vi "Dispatch Worker Mode Example(Async).vi"() -> ()   [LabVIEW 2014]
uses:
  user.lib/_NEVSTOP/JKI State Machine ++/_Support/JKISMQ/_JKISMQFGV.vi
  user.lib/_NEVSTOP/JKI State Machine ++/JKI-State-Machine-Plus.lvlib
panel:
  in  "Macro: Exit -@ Worker":bool
  in  "DoSth: DoA -@ Worker":bool
  in  "Name(\"\" to use uuid)":string="Event JKISM"
  out "State History":string
  in  "DoSth: DoA -> Worker":bool
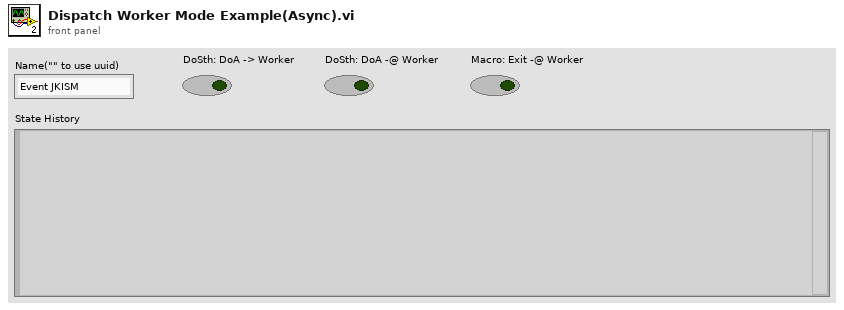
[diagram p1: front panel]
types:
  T1 = enum32{"Invalid", "Standard", "Closed", "Hidden", "Minimized", "Maximized"}
  T2 = enum32{"invalid app kind", "Development System", "Run Time System", "Student Edition", "Embedded LabVIEW", "Evaluation", "Custom"}
  T3 = cluster{"Core":cluster{"Current VI Reference":refnum<vi>, "Close Panel on Exit?":bool}, "Your Boolean data":bool, "Your string data":string}
  T4 = cluster{"Current VI Reference":refnum<vi>, "Close Panel on Exit?":bool}
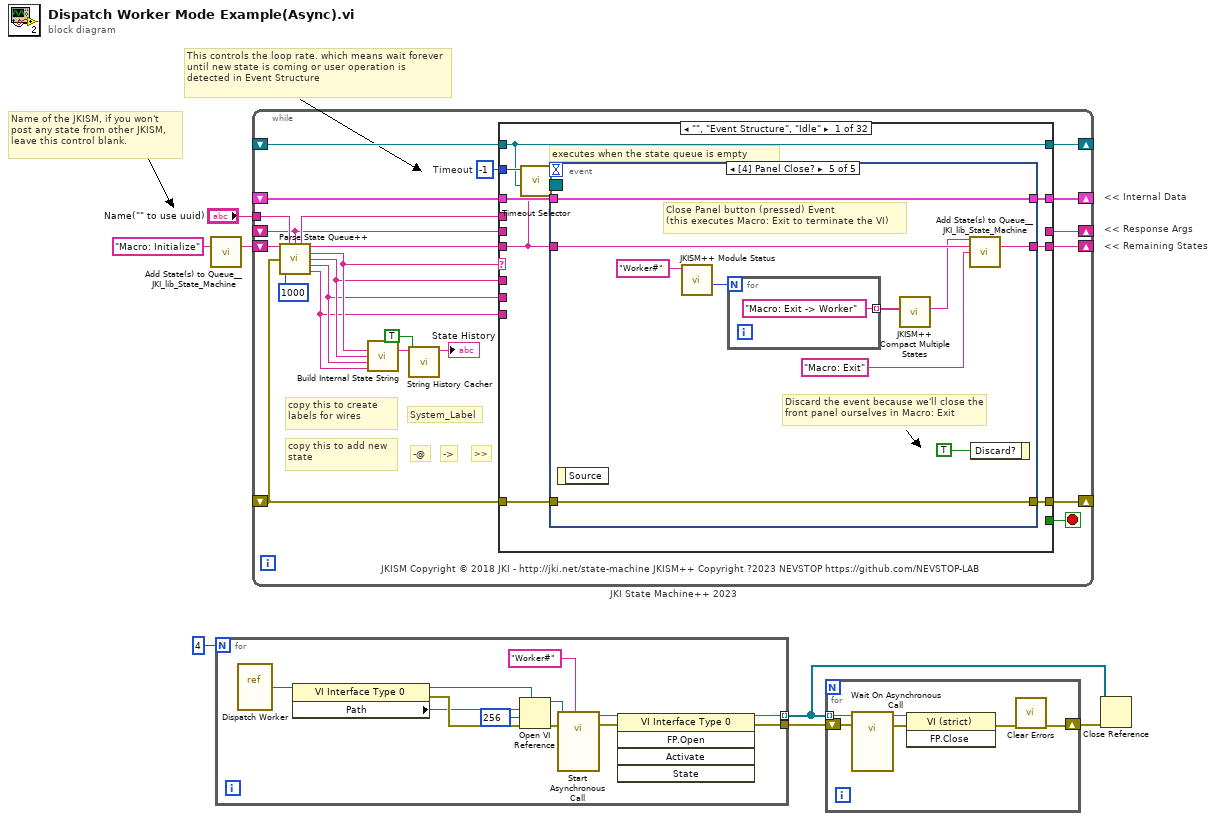
[diagram p0: block diagram]
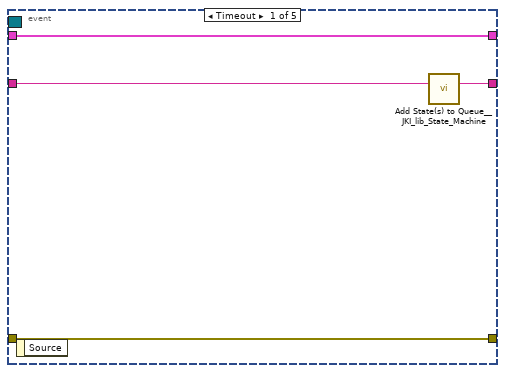
[diagram p2: hidden frame]
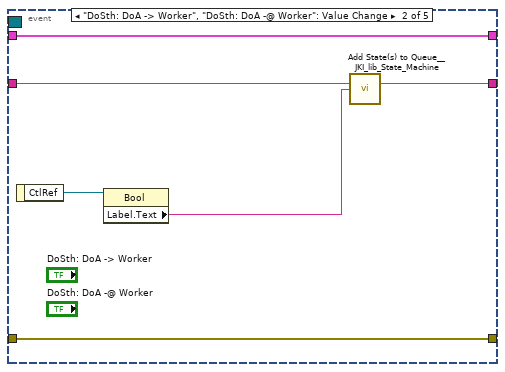
[diagram p3: hidden frame]
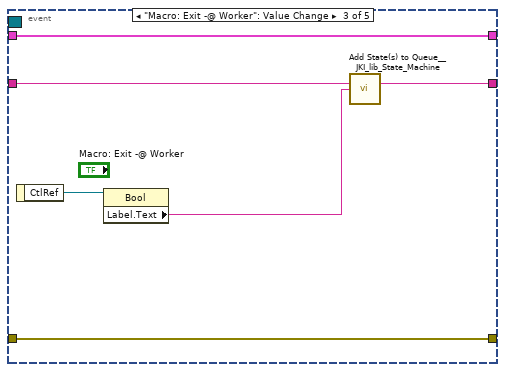
[diagram p4: hidden frame]
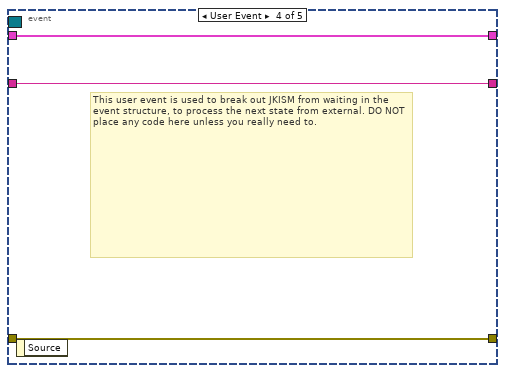
[diagram p5: hidden frame]
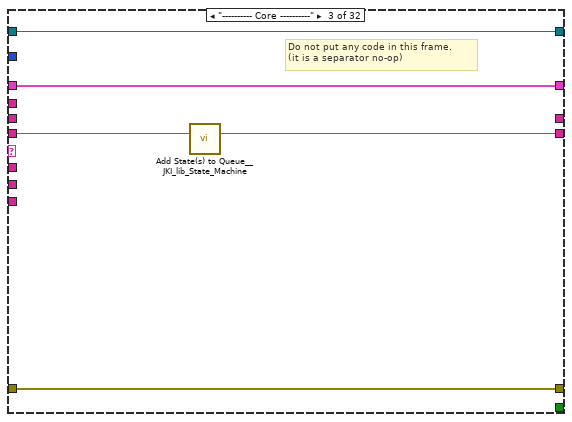
[diagram p7: hidden frame]
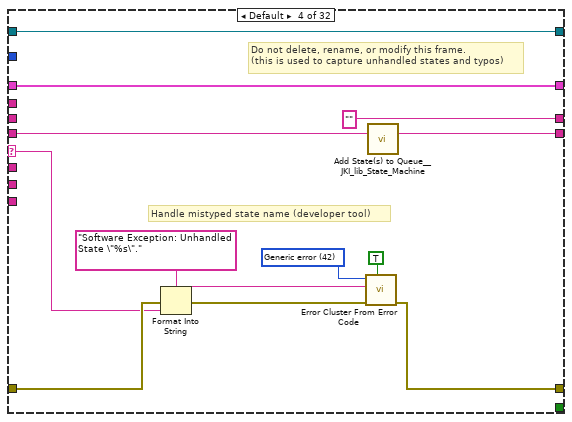
[diagram p8: hidden frame]
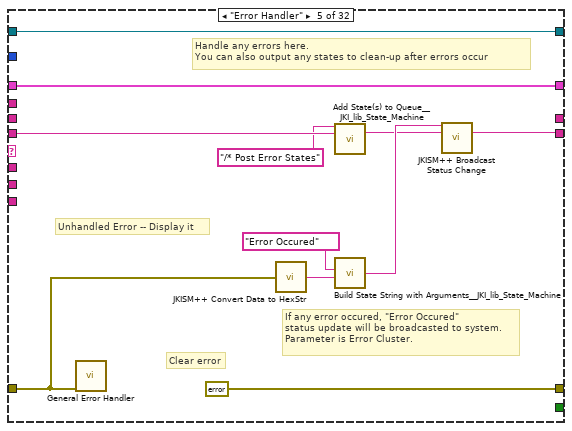
[diagram p9: hidden frame]
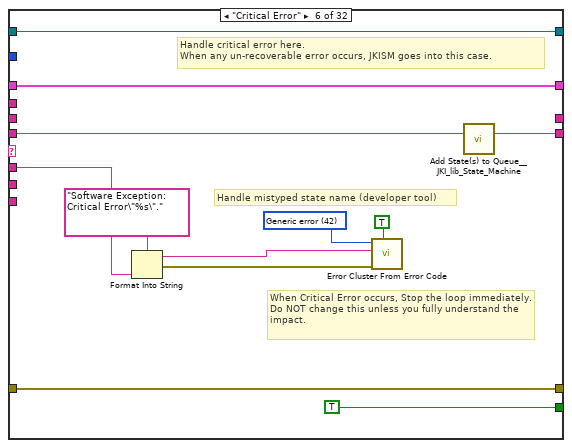
[diagram p10: hidden frame]
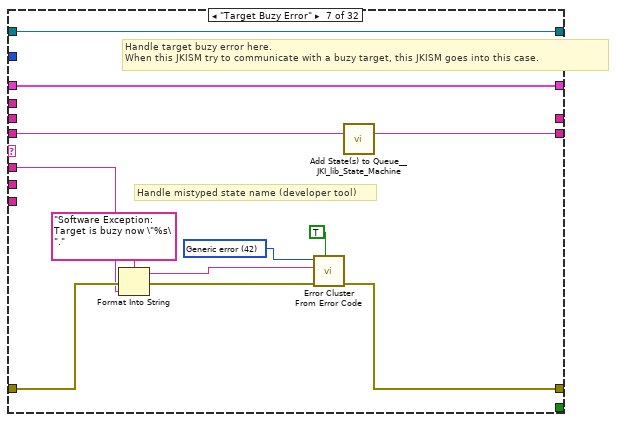
[diagram p11: hidden frame]
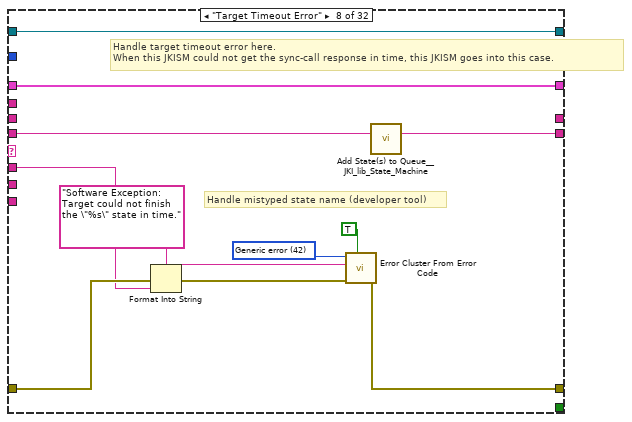
[diagram p12: hidden frame]
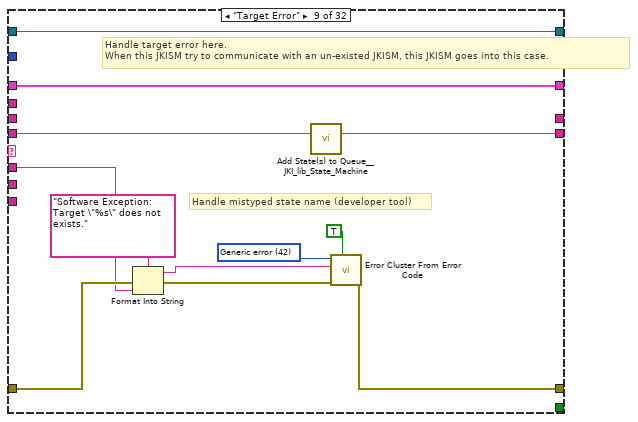
[diagram p13: hidden frame]
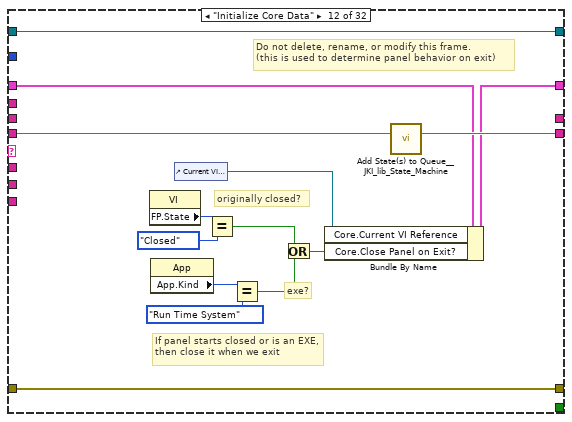
[diagram p16: hidden frame]
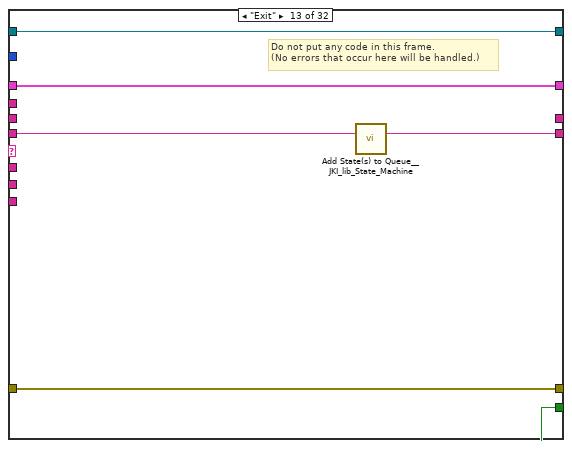
[diagram p17: hidden frame]
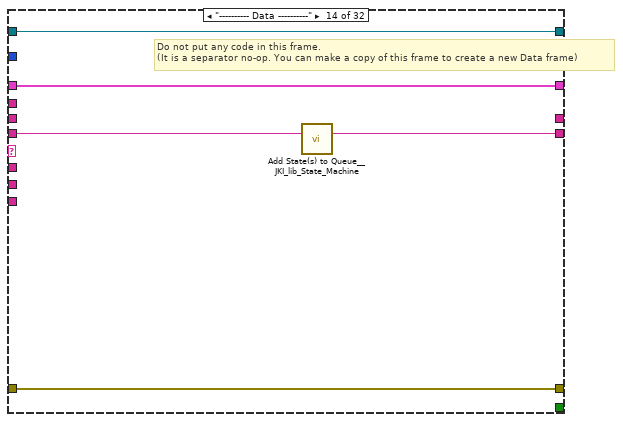
[diagram p18: hidden frame]
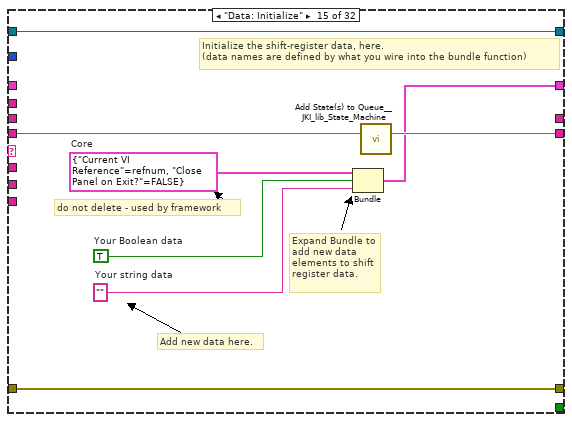
[diagram p19: hidden frame]
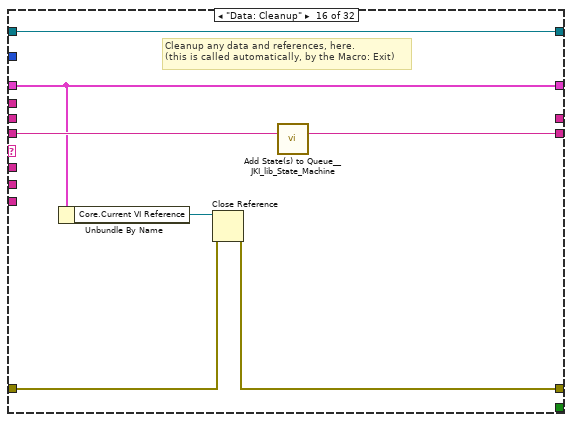
[diagram p20: hidden frame]
diagram:
  # "Name of the JKISM, if you won't post any state from other JKISM,  leave this control blank."
  # "This controls the loop rate. which means wait forever until new state is coming or user operation is detected in Event Structure"
  # "<< Internal Data"
  # "<< Response Args"
  # "<< Remaining States"
  n1 = call <vilib>:"Add State(s) to Queue__JKI_lib_State_Machine.vi"("State(s) in (\"\")"="Macro: Initialize") -> ("States Out"=w7:string)  [unwired: 14 in]
  n2 = for {
    N: 4 -> [_]
    tunnel: [w9] -> w4
    tunnel: [w10] -> w1 mode=indexing
    n3 = vi-ref "Dispatch Worker.vi"() -> (w13:refnum<vi>)
    n4 = property class="VI Interface Type 0"(reference=w13) -> (reference out=w17:refnum<vi>, error out=w15:errorcluster, "Path"=w14:path)  [unwired: 1 in]
    n5 = Open VI Reference(type specifier VI Refnum (for type only)=w17, vi path=w14, options=256, error in (no error)=w15) -> (vi reference=w16:refnum<vi>, error out=w12:errorcluster)  [unwired: 2 in]
    n6 = call-by-ref "Start Asynchronous Call"(reference=w16, error in=w12, "Name(\"\" to use uuid)"="Worker#" ("Name(\"\" to use uuid)")) -> (reference out=w11:refnum<vi>, error out=w8:errorcluster)  [unwired: 11 in]
    n7 = invoke class="VI Interface Type 0" method="FP.Open"(reference=w11, error in=w8) -> (reference out=w10:refnum<vi>, error out=w9:errorcluster)  [unwired: 3 in, 3 out]
  }
  n8 = while "JKI State Machine++ 2023" {
    shift-right: [w37] -> _
    shift-left: _ -> [w36]
    shift-right: [w40] -> _
    shift-left: _ -> [w34]
    shift-right: [w39] -> _
    shift-left: w7 -> [w41]
    tunnel: "Name(\"\" to use uuid)" -> [w29]
    shift-right: [w32] -> _
    shift-left: _ -> [w21]
    shift-right: [w31] -> _
    shift-left: _ -> [w30]
    stop <- w38 stop-if-true
    w35 = -1  # Timeout
    # "JKISM Copyright © 2018 JKI - http://jki.net/state-machine JKISM++ Copyright ?2023 NEVSTOP https://github.com/NEVSTOP-LAB"
    # "copy this to add new state"
    # ">>"
    # "->"
    # "-@"
    # "copy this to create labels for wires"
    # "System_Label"
    n9 = call "Parse State Queue++.vi"("State Queue"=w41, "Name(\"\" to use uuid)"=w29, "Response Arguments"=w21, "Error In (no error)"=w34, "Response Timeout(5000ms)"=1000 ("Response Timeout(1000ms)")) -> ("Name Used"=w22:string, "Remaining States"=w42:string, "Current State"=w26:string, "Arguments"=w25:string, "Argument - State"=w24:string, "From Who"=w23:string)  [unwired: 5 in]
    n10 = call "Build Internal State String.vi"("State"=w26, "Arguments (\"\")"=w25, "Arg-State (\"\")"=w24, "Source (\"\")"=w23) -> ("State with Arguments"=w27:string)  [unwired: 11 in]
    n11 = call "String History Cacher.vi"("Include Timestamp(F)"=TRUE, "String"=w27) -> ("String Cache"=→"State History":string)  [unwired: 9 in]
    n12 = case shown="\"\", \"Event Structure\", \"Idle\"" w26 {
      selector: w26 -> [_ _ _ w93 _ _ _ _ _ _ _ _ _ _ _ _ _ _ _ _ _ _ _ _ _ _ _ _ _ _ _ _]
      tunnel: w42 -> [w43 w84 w90 w97 w114 w124 w127 w144 w156 w165 w169 w184 w190 w195 w203 w210 w215 w221 w225 w231 w236 w243 w259 w329 w335 w346 w349 w354 w360 w368 w374 w380]
      tunnel: w25 -> [_ _ _ _ _ w117 w129 w140 w152 _ _ _ _ _ _ _ _ _ _ _ _ w238 w253 _ _ _ _ _ w357 _ _ _]
      tunnel: w36 -> [w50 w83 w87 w95 w112 w125 w131 w142 w154 w164 w168 w177 w188 w192 _ w205 w212 w220 w224 w228 w234 w241 w255 w326 w332 w343 w348 w353 w359 w365 w371 w377]
      tunnel: [w49 w85 w88 w99 errorcluster {"status"=FALSE, "code"=0, "source"=""} ("error out") w126 w134 w146 w158 w166 w170 w181 w187 w193 w200 w206 w213 w216 w223 w229 w233 w239 w256 w327 w333 w344 w350 w355 w361 w366 w372 w378] -> w40
      tunnel: w34 -> [w48 w85 w88 w98 w104 w126 w133 w145 w157 w166 w170 w181 w187 w193 w200 w207 w213 _ w226 w229 w233 w240 w257 w327 w333 w344 w350 w355 w361 w366 w372 w378]
      tunnel: [w51 w84 w89 w96 w105 w123 w132 w143 w155 w165 w169 w183 w189 w194 w202 w209 w214 w221 w225 w230 w235 w242 w258 w328 w334 w345 w349 w354 w360 w367 w373 w379] -> w39
      tunnel: [_ _ _ _ _ TRUE _ _ _ _ _ _ TRUE _ _ _ _ _ _ _ _ _ _ _ _ _ _ _ _ _ _ _] -> w38
      tunnel: [w47 w83 w87 w95 w112 w125 w131 w142 w154 w164 w168 w182 w188 w192 w201 w205 w212 w220 w224 w228 w234 w241 w255 w326 w332 w343 w348 w353 w359 w365 w371 w377] -> w37
      tunnel: w35 -> [w46 _ _ _ _ _ _ _ _ _ _ _ _ _ _ _ _ _ _ _ _ _ _ _ _ _ _ _ _ _ _ _]
      tunnel: w23 -> [_ _ _ _ _ _ _ _ _ _ _ _ _ _ _ _ _ _ _ _ _ _ _ _ _ _ _ _ _ _ _ _]
      tunnel: w24 -> [_ _ _ _ _ _ _ _ _ _ _ _ _ _ _ _ _ _ _ _ _ _ _ _ _ _ _ _ _ _ _ _]
      tunnel: [_ _ _ "" _ _ _ _ _ _ _ _ _ _ _ _ _ _ _ _ _ _ _ _ _ _ _ "API1 Response" w356 _ "DoA Finished" "DoB Finished"] -> w32
      tunnel: [w45 w82 w86 w91 w110 w115 w128 w139 w151 w163 w167 w171 w185 w191 w196 w204 w211 w219 w222 w227 w232 w237 w252 w325 w330 w336 w347 w352 w358 w364 w370 w376] -> w31
      tunnel: w30 -> [w45 w82 w86 w91 w110 w115 w128 w139 w151 w163 w167 w171 w185 w191 w196 w204 w211 _ w222 w227 w232 w237 w252 w325 w330 w336 w347 w352 w358 w364 w370 w376]
      tunnel: w22 -> [_ _ _ _ _ _ _ _ _ _ _ _ _ _ _ _ _ w218 _ _ _ _ _ _ _ _ _ _ _ _ _ _]
      tunnel: w21 -> [_ _ _ _ _ _ _ _ _ _ _ _ _ _ _ _ _ _ _ _ _ _ _ _ _ _ _ _ _ _ _ _]
      frame "", "Event Structure", "Idle" {
        # "executes when the state queue is empty"
        n13 = call "Timeout Selector.vi"("Remaining States"=w43, "Timeout Expected"=w46) -> ("Timeout"=w44:i32)  [unwired: 5 in]
        n14 = event shown="[4] Panel Close?" {
          selector: w45 -> [_ _ _ _ _]
          dyn-events: _ -> [_ _ _ _ _]
          timeout: w44 -> [_ _ _ _ _]
          tunnel: w43 -> [w55 w59 w65 w69 w80]
          tunnel: [w54 w58 w64 w69 w79] -> w51
          tunnel: w50 -> [w52 w60 w66 w70 w77]
          tunnel: [w53 w61 w67 w68 w78] -> w49
          tunnel: w48 -> [w53 w61 w67 w68 w78]
          tunnel: [w52 w60 w66 w70 w77] -> w47
          event Timeout {
            n15 = event-data() -> ()  [unwired: 1 in, 1 out]
            n16 = call <vilib>:"Add State(s) to Queue__JKI_lib_State_Machine.vi"("State(s) in (\"\")"=w55) -> ("States Out"=w54:string)  [unwired: 14 in]
          }
          event "DoSth: DoA -> Worker", "DoSth: DoA -@ Worker": Value Change {
            n17 = event-data() -> ("CtlRef"=w57:refnum<vi>)  [unwired: 1 in]
            n18 = property class="Bool"(reference=w57) -> ("Label.Text"=w56:string)  [unwired: 1 in, 2 out]
            n19 = call <vilib>:"Add State(s) to Queue__JKI_lib_State_Machine.vi"("State(s) in (\"\")"=w59, "State(s) at Back (\"\")"=w56) -> ("States Out"=w58:string)  [unwired: 13 in]
          }
          event "Macro: Exit -@ Worker": Value Change {
            n20 = event-data() -> ("CtlRef"=w63:refnum<vi>)  [unwired: 1 in]
            n21 = property class="Bool"(reference=w63) -> ("Label.Text"=w62:string)  [unwired: 1 in, 2 out]
            n22 = call <vilib>:"Add State(s) to Queue__JKI_lib_State_Machine.vi"("State(s) in (\"\")"=w65, "State(s) at Back (\"\")"=w62) -> ("States Out"=w64:string)  [unwired: 13 in]
          }
          event User Event {
            # "This user event is used to break out JKISM from waiting in the event structure, to process the next state from external. DO NOT place any code here unless you really need to."
            n23 = event-data() -> ()  [unwired: 1 in, 1 out]
          }
          event Panel Close? {
            # "Discard the event because we'll close the front panel ourselves in Macro: Exit"
            # "Close Panel button (pressed) Event\n(this executes Macro: Exit to terminate the VI)"
            n24 = event-data() -> ()  [unwired: 1 in, 1 out]
            n25 = call "JKISM++ Module Status.vi"("JKISM Name"="Worker#" ("Name(\"\" to use uuid)")) -> ("#AsWorker"=w71:i32)  [unwired: 6 in, 4 out]
            n26 = for {
              N: w71 -> [_]
              tunnel: ["Macro: Exit -> Worker"] -> w75 mode=indexing
            }
            n27 = call "JKISM++ Compact Multiple States.vi"("States in Lines"=w75) -> ("States"=w72:string)  [unwired: 9 in]
            n28 = call <vilib>:"Add State(s) to Queue__JKI_lib_State_Machine.vi"("State(s) in Front (\"\")"=w72, "State(s) in (\"\")"=w80, "State(s) at Back (\"\")"="Macro: Exit") -> ("States Out"=w79:string)  [unwired: 12 in]
            n29 = event-data("Discard?"=TRUE) -> ()  [unwired: 1 in, 1 out]
          }
        }
      }
      frame "JKISM++ Documentation" {
        # "JKISM++ Documentation"
        # "State Syntax:\nStateCategory: State >> Argument -@ JKISMName\nStateCategory: State >> Argument -> JKISMName\n\nLine Terminator: Line feed"
        # "Commenting:\nTo add a comment use \"//\" or \"#\" and all text to the right will be ignored\nCommenting Example:\nUI: Initialize // This initializes the UI\n# This whole line is a comment\n// Another comment line"
      }
      frame "---------- Core ----------" {
        # "Do not put any code in this frame.\n(it is a separator no-op)"
        n30 = call <vilib>:"Add State(s) to Queue__JKI_lib_State_Machine.vi"("State(s) in (\"\")"=w90) -> ("States Out"=w89:string)  [unwired: 14 in]
      }
      frame Default {
        w102 = 42 items=["No error", "Argument error", "Memory is full", "Out of zone", "End of file", "File already open", "Generic file I/O error", "File not found", "File permission error", "Disk is full", "Duplicate path", "Too many files open", "System feature not enabled", "Resource file not found", "Cannot add resource", "Resource not found", "Image not found", "Image memory error", "Pen does not exist", "Config type invalid", "Config token not found", "Config parse error", "Config memory error", "Bad external code format", "Bad external code offset", "External code not present", "Null window", "Destroy window error", "Null menu", "Print aborted", "Bad print record", "Print driver error", "Windows error during printing", "Memory error during printing", "Print dialog error", "Generic print error", "Invalid device refnum", "Device not found", "Device parameter error", "Device unit error", "Cannot open device", "Device call aborted", "Generic error", "Cancelled by user", "Object ID too low", "Object ID too high", "Object not in heap", "Unknown heap", "Unknown object (invalid DefProc)", "Unknown object (DefProc not in table)", "Message out of range", "Invalid (null) method", "Unknown message", "Manager call not supported", "Bad address", "Network operation in progress", "Network operation timed out", "Connection is busy", "Network attribute not supported", "Network error", "Address in use", "System out of memory", "Connection aborted", "Connection refused", "Not connected", "Already connected", "Connection closed", "Initialization error (interapplication manager)", "Bad occurrence", "Wait on unbound occurrence handler", "Occurrence queue overflow", "Datalog type conflict", "Unused", "Unrecognized type (interapplication manager)", "Memory corrupt", "Failed to make temporary DLL", "Old CIN version", "Drag socket not found", "Failed to load drop-object", "Failed to register OLE object", "Failed to release OLE object", "Format specifier type mismatch", "Unknown format specifier", "Too few format specifiers", "Too many format specifiers", "Scan failed", "Newer CIN version", "Error converting to variant", "Runtime menu error", "Password tampered", "Variant attribute not found", "Incompatible variant data type", "Event data is not available", "Event Store is not present", "Occurrence is not found", "Event Queue is not created", "Event info is not available", "Refnum passed is NULL", "Error retrieving Class GUID", "Error retrieving CoClass GUID", "Error retrieving TypeLib GUID.", "Bad built application magic bytes.", "Specific driver is different from the specific driver associated with the Logical Name.", "There is no session opened to the class driver.", "Max Error", "MAX - Error with config objects", "MAX - Error loading configuration", "MAX - Group not supported"]
        # "Do not delete, rename, or modify this frame.\n(this is used to capture unhandled states and typos)"
        # "Handle mistyped state name (developer tool)"
        n31 = Format Into String(format string="Software Exception: Unhandled State \"%s\"." ("message"), error in=w98, w93) -> (resulting string=w101:string, error out=w100:errorcluster)  [unwired: 1 in]
        n32 = call <vilib>:"Error Cluster From Error Code.vi"("show call chain? (False)"=TRUE, "error in (no error)"=w100, "error message (\"\")"=w101, "error code (0)"=w102) -> ("error out"=w99:errorcluster)  [unwired: 5 in]
        n33 = call <vilib>:"Add State(s) to Queue__JKI_lib_State_Machine.vi"("State(s) in (\"\")"=w97) -> ("States Out"=w96:string)  [unwired: 14 in]
      }
      frame "Error Handler" {
        # "If any error occured, \"Error Occured\" \nstatus update will be broadcasted to system.\nParameter is Error Cluster."
        # "Unhandled Error -- Display it"
        # "Handle any errors here.\nYou can also output any states to clean-up after errors occur"
        # "Clear error"
        n34 = call <vilib>:"General Error Handler.vi"("error in (no error)"=w104) -> ()  [unwired: 10 in, 5 out]
        n35 = call "JKISM++ Convert Data to HexStr.vi"("Variant"=w104) -> ("HEX String (0-9,A-F)"=w108:string)  [unwired: 8 in]
        n36 = call <vilib>:"Add State(s) to Queue__JKI_lib_State_Machine.vi"("State(s) in Front (\"\")"="/* Post Error States", "State(s) in (\"\")"=w114) -> ("States Out"=w106:string)  [unwired: 13 in]
        n37 = call <vilib>:"Build State String with Arguments__JKI_lib_State_Machine.vi"("Arguments (\"\")"=w108, "State"="Error Occured" ("Status with Arguments")) -> ("State with Arguments"=w107:string)  [unwired: 4 in]
        n38 = call "JKISM++ Broadcast Status Change.vi"("Status with Arguments"=w107, "State(s) in (\"\")"=w106) -> ("States Out"=w105:string)  [unwired: 13 in]
      }
      frame "Critical Error" {
        w121 = 42 items=["No error", "Argument error", "Memory is full", "Out of zone", "End of file", "File already open", "Generic file I/O error", "File not found", "File permission error", "Disk is full", "Duplicate path", "Too many files open", "System feature not enabled", "Resource file not found", "Cannot add resource", "Resource not found", "Image not found", "Image memory error", "Pen does not exist", "Config type invalid", "Config token not found", "Config parse error", "Config memory error", "Bad external code format", "Bad external code offset", "External code not present", "Null window", "Destroy window error", "Null menu", "Print aborted", "Bad print record", "Print driver error", "Windows error during printing", "Memory error during printing", "Print dialog error", "Generic print error", "Invalid device refnum", "Device not found", "Device parameter error", "Device unit error", "Cannot open device", "Device call aborted", "Generic error", "Cancelled by user", "Object ID too low", "Object ID too high", "Object not in heap", "Unknown heap", "Unknown object (invalid DefProc)", "Unknown object (DefProc not in table)", "Message out of range", "Invalid (null) method", "Unknown message", "Manager call not supported", "Bad address", "Network operation in progress", "Network operation timed out", "Connection is busy", "Network attribute not supported", "Network error", "Address in use", "System out of memory", "Connection aborted", "Connection refused", "Not connected", "Already connected", "Connection closed", "Initialization error (interapplication manager)", "Bad occurrence", "Wait on unbound occurrence handler", "Occurrence queue overflow", "Datalog type conflict", "Unused", "Unrecognized type (interapplication manager)", "Memory corrupt", "Failed to make temporary DLL", "Old CIN version", "Drag socket not found", "Failed to load drop-object", "Failed to register OLE object", "Failed to release OLE object", "Format specifier type mismatch", "Unknown format specifier", "Too few format specifiers", "Too many format specifiers", "Scan failed", "Newer CIN version", "Error converting to variant", "Runtime menu error", "Password tampered", "Variant attribute not found", "Incompatible variant data type", "Event data is not available", "Event Store is not present", "Occurrence is not found", "Event Queue is not created", "Event info is not available", "Refnum passed is NULL", "Error retrieving Class GUID", "Error retrieving CoClass GUID", "Error retrieving TypeLib GUID.", "Bad built application magic bytes.", "Specific driver is different from the specific driver associated with the Logical Name.", "There is no session opened to the class driver.", "Max Error", "MAX - Error with config objects", "MAX - Error loading configuration", "MAX - Group not supported"]
        # "Handle critical error here.\nWhen any un-recoverable error occurs, JKISM goes into this case."
        # "When Critical Error occurs, Stop the loop immediately. Do NOT change this unless you fully understand the impact."
        # "Handle mistyped state name (developer tool)"
        n39 = Format Into String(format string="Software Exception: Critical Error\"%s\"." ("message"), w117) -> (resulting string=w120:string, error out=w119:errorcluster)  [unwired: 2 in]
        n40 = call <vilib>:"Error Cluster From Error Code.vi"("show call chain? (False)"=TRUE, "error in (no error)"=w119, "error message (\"\")"=w120, "error code (0)"=w121) -> ()  [unwired: 5 in, 1 out]
        n41 = call <vilib>:"Add State(s) to Queue__JKI_lib_State_Machine.vi"("State(s) in (\"\")"=w124) -> ("States Out"=w123:string)  [unwired: 14 in]
      }
      frame "Target Buzy Error" {
        w137 = 42 items=["No error", "Argument error", "Memory is full", "Out of zone", "End of file", "File already open", "Generic file I/O error", "File not found", "File permission error", "Disk is full", "Duplicate path", "Too many files open", "System feature not enabled", "Resource file not found", "Cannot add resource", "Resource not found", "Image not found", "Image memory error", "Pen does not exist", "Config type invalid", "Config token not found", "Config parse error", "Config memory error", "Bad external code format", "Bad external code offset", "External code not present", "Null window", "Destroy window error", "Null menu", "Print aborted", "Bad print record", "Print driver error", "Windows error during printing", "Memory error during printing", "Print dialog error", "Generic print error", "Invalid device refnum", "Device not found", "Device parameter error", "Device unit error", "Cannot open device", "Device call aborted", "Generic error", "Cancelled by user", "Object ID too low", "Object ID too high", "Object not in heap", "Unknown heap", "Unknown object (invalid DefProc)", "Unknown object (DefProc not in table)", "Message out of range", "Invalid (null) method", "Unknown message", "Manager call not supported", "Bad address", "Network operation in progress", "Network operation timed out", "Connection is busy", "Network attribute not supported", "Network error", "Address in use", "System out of memory", "Connection aborted", "Connection refused", "Not connected", "Already connected", "Connection closed", "Initialization error (interapplication manager)", "Bad occurrence", "Wait on unbound occurrence handler", "Occurrence queue overflow", "Datalog type conflict", "Unused", "Unrecognized type (interapplication manager)", "Memory corrupt", "Failed to make temporary DLL", "Old CIN version", "Drag socket not found", "Failed to load drop-object", "Failed to register OLE object", "Failed to release OLE object", "Format specifier type mismatch", "Unknown format specifier", "Too few format specifiers", "Too many format specifiers", "Scan failed", "Newer CIN version", "Error converting to variant", "Runtime menu error", "Password tampered", "Variant attribute not found", "Incompatible variant data type", "Event data is not available", "Event Store is not present", "Occurrence is not found", "Event Queue is not created", "Event info is not available", "Refnum passed is NULL", "Error retrieving Class GUID", "Error retrieving CoClass GUID", "Error retrieving TypeLib GUID.", "Bad built application magic bytes.", "Specific driver is different from the specific driver associated with the Logical Name.", "There is no session opened to the class driver.", "Max Error", "MAX - Error with config objects", "MAX - Error loading configuration", "MAX - Group not supported"]
        # "Handle target buzy error here.\nWhen this JKISM try to communicate with a buzy target, this JKISM goes into this case."
        # "Handle mistyped state name (developer tool)"
        n42 = Format Into String(format string="Software Exception: Target is buzy now \"%s\"." ("message"), error in=w133, w129) -> (resulting string=w136:string, error out=w135:errorcluster)  [unwired: 1 in]
        n43 = call <vilib>:"Error Cluster From Error Code.vi"("show call chain? (False)"=TRUE, "error in (no error)"=w135, "error message (\"\")"=w136, "error code (0)"=w137) -> ("error out"=w134:errorcluster)  [unwired: 5 in]
        n44 = call <vilib>:"Add State(s) to Queue__JKI_lib_State_Machine.vi"("State(s) in (\"\")"=w127) -> ("States Out"=w132:string)  [unwired: 14 in]
      }
      frame "Target Timeout Error" {
        w149 = 42 items=["No error", "Argument error", "Memory is full", "Out of zone", "End of file", "File already open", "Generic file I/O error", "File not found", "File permission error", "Disk is full", "Duplicate path", "Too many files open", "System feature not enabled", "Resource file not found", "Cannot add resource", "Resource not found", "Image not found", "Image memory error", "Pen does not exist", "Config type invalid", "Config token not found", "Config parse error", "Config memory error", "Bad external code format", "Bad external code offset", "External code not present", "Null window", "Destroy window error", "Null menu", "Print aborted", "Bad print record", "Print driver error", "Windows error during printing", "Memory error during printing", "Print dialog error", "Generic print error", "Invalid device refnum", "Device not found", "Device parameter error", "Device unit error", "Cannot open device", "Device call aborted", "Generic error", "Cancelled by user", "Object ID too low", "Object ID too high", "Object not in heap", "Unknown heap", "Unknown object (invalid DefProc)", "Unknown object (DefProc not in table)", "Message out of range", "Invalid (null) method", "Unknown message", "Manager call not supported", "Bad address", "Network operation in progress", "Network operation timed out", "Connection is busy", "Network attribute not supported", "Network error", "Address in use", "System out of memory", "Connection aborted", "Connection refused", "Not connected", "Already connected", "Connection closed", "Initialization error (interapplication manager)", "Bad occurrence", "Wait on unbound occurrence handler", "Occurrence queue overflow", "Datalog type conflict", "Unused", "Unrecognized type (interapplication manager)", "Memory corrupt", "Failed to make temporary DLL", "Old CIN version", "Drag socket not found", "Failed to load drop-object", "Failed to register OLE object", "Failed to release OLE object", "Format specifier type mismatch", "Unknown format specifier", "Too few format specifiers", "Too many format specifiers", "Scan failed", "Newer CIN version", "Error converting to variant", "Runtime menu error", "Password tampered", "Variant attribute not found", "Incompatible variant data type", "Event data is not available", "Event Store is not present", "Occurrence is not found", "Event Queue is not created", "Event info is not available", "Refnum passed is NULL", "Error retrieving Class GUID", "Error retrieving CoClass GUID", "Error retrieving TypeLib GUID.", "Bad built application magic bytes.", "Specific driver is different from the specific driver associated with the Logical Name.", "There is no session opened to the class driver.", "Max Error", "MAX - Error with config objects", "MAX - Error loading configuration", "MAX - Group not supported"]
        # "Handle target timeout error here.\nWhen this JKISM could not get the sync-call response in time, this JKISM goes into this case."
        # "Handle mistyped state name (developer tool)"
        n45 = Format Into String(format string="Software Exception: Target could not finish the \"%s\" state in time." ("message"), error in=w145, w140) -> (resulting string=w148:string, error out=w147:errorcluster)  [unwired: 1 in]
        n46 = call <vilib>:"Error Cluster From Error Code.vi"("show call chain? (False)"=TRUE, "error in (no error)"=w147, "error message (\"\")"=w148, "error code (0)"=w149) -> ("error out"=w146:errorcluster)  [unwired: 5 in]
        n47 = call <vilib>:"Add State(s) to Queue__JKI_lib_State_Machine.vi"("State(s) in (\"\")"=w144) -> ("States Out"=w143:string)  [unwired: 14 in]
      }
      frame "Target Error" {
        w161 = 42 items=["No error", "Argument error", "Memory is full", "Out of zone", "End of file", "File already open", "Generic file I/O error", "File not found", "File permission error", "Disk is full", "Duplicate path", "Too many files open", "System feature not enabled", "Resource file not found", "Cannot add resource", "Resource not found", "Image not found", "Image memory error", "Pen does not exist", "Config type invalid", "Config token not found", "Config parse error", "Config memory error", "Bad external code format", "Bad external code offset", "External code not present", "Null window", "Destroy window error", "Null menu", "Print aborted", "Bad print record", "Print driver error", "Windows error during printing", "Memory error during printing", "Print dialog error", "Generic print error", "Invalid device refnum", "Device not found", "Device parameter error", "Device unit error", "Cannot open device", "Device call aborted", "Generic error", "Cancelled by user", "Object ID too low", "Object ID too high", "Object not in heap", "Unknown heap", "Unknown object (invalid DefProc)", "Unknown object (DefProc not in table)", "Message out of range", "Invalid (null) method", "Unknown message", "Manager call not supported", "Bad address", "Network operation in progress", "Network operation timed out", "Connection is busy", "Network attribute not supported", "Network error", "Address in use", "System out of memory", "Connection aborted", "Connection refused", "Not connected", "Already connected", "Connection closed", "Initialization error (interapplication manager)", "Bad occurrence", "Wait on unbound occurrence handler", "Occurrence queue overflow", "Datalog type conflict", "Unused", "Unrecognized type (interapplication manager)", "Memory corrupt", "Failed to make temporary DLL", "Old CIN version", "Drag socket not found", "Failed to load drop-object", "Failed to register OLE object", "Failed to release OLE object", "Format specifier type mismatch", "Unknown format specifier", "Too few format specifiers", "Too many format specifiers", "Scan failed", "Newer CIN version", "Error converting to variant", "Runtime menu error", "Password tampered", "Variant attribute not found", "Incompatible variant data type", "Event data is not available", "Event Store is not present", "Occurrence is not found", "Event Queue is not created", "Event info is not available", "Refnum passed is NULL", "Error retrieving Class GUID", "Error retrieving CoClass GUID", "Error retrieving TypeLib GUID.", "Bad built application magic bytes.", "Specific driver is different from the specific driver associated with the Logical Name.", "There is no session opened to the class driver.", "Max Error", "MAX - Error with config objects", "MAX - Error loading configuration", "MAX - Group not supported"]
        # "Handle target error here.\nWhen this JKISM try to communicate with an un-existed JKISM, this JKISM goes into this case."
        # "Handle mistyped state name (developer tool)"
        n48 = Format Into String(format string="Software Exception: Target \"%s\" does not exists." ("message"), error in=w157, w152) -> (resulting string=w160:string, error out=w159:errorcluster)  [unwired: 1 in]
        n49 = call <vilib>:"Add State(s) to Queue__JKI_lib_State_Machine.vi"("State(s) in (\"\")"=w156) -> ("States Out"=w155:string)  [unwired: 14 in]
        n50 = call <vilib>:"Error Cluster From Error Code.vi"("show call chain? (False)"=TRUE, "error in (no error)"=w159, "error message (\"\")"=w160, "error code (0)"=w161) -> ("error out"=w158:errorcluster)  [unwired: 5 in]
      }
      frame "Async Response", "Response" {
        # "Handle Async-call Response (\"Async Response\" for ->)"
        # "Handle Sync-call Response (\"Response\" for @)"
        # "After Message is excuted, JKISM+ goes to this state for recieve the response. \n    For Async Message(->), \"Async Response\" is used. This JKISM will goes to \"Async Message Posted\" immediately and recieve the \"Async Response\" after the callee finishes the message.\n    For Sync Message(@),  This JKISM will wait until the message is done and immidieatly goes to \"Response\""
      }
      frame "Async Message Posted" {
        # "Handle post action for async message (->)."
        # "After Async Message is posted (->), JKISM+ goes to this state for post-action. You can use Argument - State to tell which Async Message is called."
      }
      frame "Initialize Core Data" {
        # "Do not delete, rename, or modify this frame.\n(this is used to determine panel behavior on exit)"
        # "originally closed?"
        # "exe?"
        # "If panel starts closed or is an EXE, then close it when we exit"
        n51 = property class="VI"() -> ("FP.State"=w174:T1)  [unwired: 2 in, 2 out]
        n52 = property class="App"() -> ("App.Kind"=w180:T2)  [unwired: 2 in, 2 out]
        n53 = control-ref of="Current VI Reference"() -> (w175:refnum<vi>)
        n54 = Equal?(x=w174, y=T1."Closed" ("Front Panel Window:State")) -> (x = y?=w172:bool)
        n55 = Equal?(x=w180, y=T2."Run Time System" ("Application:Kind")) -> (x = y?=w178:bool)
        n56 = Or(x=w172, y=w178) -> (x .or. y?=w176:bool)
        n57 = Bundle By Name(cluster=w177, "Core.Current VI Reference"=w175, "Core.Close Panel on Exit?"=w176) -> (w182:T3)
        n58 = call <vilib>:"Add State(s) to Queue__JKI_lib_State_Machine.vi"("State(s) in (\"\")"=w184) -> ("States Out"=w183:string)  [unwired: 14 in]
      }
      frame "Exit" {
        # "Do not put any code in this frame.\n(No errors that occur here will be handled.)"
        n59 = call <vilib>:"Add State(s) to Queue__JKI_lib_State_Machine.vi"("State(s) in (\"\")"=w190) -> ("States Out"=w189:string)  [unwired: 14 in]
      }
      frame "---------- Data ----------" {
        # "Do not put any code in this frame.\n(It is a separator no-op. You can make a copy of this frame to create a new Data frame)"
        n60 = call <vilib>:"Add State(s) to Queue__JKI_lib_State_Machine.vi"("State(s) in (\"\")"=w195) -> ("States Out"=w194:string)  [unwired: 14 in]
      }
      frame "Data: Initialize" {
        w197 = T4 {"Current VI Reference"=refnum, "Close Panel on Exit?"=FALSE}  # Core
        w199 = TRUE  # Your Boolean data
        w198 = ""  # Your string data
        # "do not delete - used by framework"
        # "Expand Bundle to add new data elements to shift register data."
        # "Add new data here."
        # "Initialize the shift-register data, here.\n(data names are defined by what you wire into the bundle function)"
        n61 = Bundle("Core"=w197, "Your Boolean data"=w199, "Your string data"=w198) -> (w201:T3)  [unwired: 1 in]
        n62 = call <vilib>:"Add State(s) to Queue__JKI_lib_State_Machine.vi"("State(s) in (\"\")"=w203) -> ("States Out"=w202:string)  [unwired: 14 in]
      }
      frame "Data: Cleanup" {
        # "Cleanup any data and references, here.\n(this is called automatically, by the Macro: Exit)"
        n63 = Unbundle By Name(w205) -> ("Core.Current VI Reference"=w208:refnum<vi>)
        n64 = Close Reference(reference=w208, error in (no error)=w207) -> (error out=w206:errorcluster)
        n65 = call <vilib>:"Add State(s) to Queue__JKI_lib_State_Machine.vi"("State(s) in (\"\")"=w210) -> ("States Out"=w209:string)  [unwired: 14 in]
      }
      frame "---------- Events ----------" {
        # "Do not put any code in this frame.\n(It is a separator no-op. You can make a copy of this frame to create a new UI frame)"
        n66 = call <vilib>:"Add State(s) to Queue__JKI_lib_State_Machine.vi"("State(s) in (\"\")"=w215) -> ("States Out"=w214:string)  [unwired: 14 in]
      }
      frame "Events: Register" {
        # "Register message event to break Waiting in Event structure."
        n67 = call "JKISM++ Get New State Notifier Event.vi"("Name(\"\" to use uuid) in"=w218) -> ("Error out"=w216:errorcluster, "New State Notifier Event"=w217:refnum<user-event>)  [unwired: 9 in]
        n68 = register-events(w217) -> (reference out=w219:refnum<event-registration>)  [unwired: 2 in, 1 out]
      }
      frame "Events: Unregister" {
        n69 = Unregister For Events(event registration refnum=w222, error in=w226) -> (error out=w223:errorcluster)
      }
      frame "---------- UI ----------" {
        # "Do not put any code in this frame.\n(It is a separator no-op. You can make a copy of this frame to create a new UI frame)"
        n70 = call <vilib>:"Add State(s) to Queue__JKI_lib_State_Machine.vi"("State(s) in (\"\")"=w231) -> ("States Out"=w230:string)  [unwired: 14 in]
      }
      frame "UI: Initialize" {
        # "Initialize the User Interface, here.\n(this is called automatically, by the Macro: Init)"
        n71 = call <vilib>:"Add State(s) to Queue__JKI_lib_State_Machine.vi"("State(s) in (\"\")"=w236) -> ("States Out"=w235:string)  [unwired: 14 in]
      }
      frame "UI: Cursor Set" {
        # "Argument"
        # "Set and Unset Cursor Busy.\n(Usage: \"UI: Cursor Set >> Busy|Idle\")"
        n72 = disable-structure shown="TARGET_TYPE!=Windows" {
          disable-tunnel: w240 -> [w246 w251]
          disable-tunnel: [w245 w251] -> w239
          disable-tunnel: w238 -> [w244 _]
          frame condition #0 (active) {
            n73 = case shown="\"Idle\", Default" w244 {
              tunnel: w246 -> [w248 w250]
              tunnel: [w247 w249] -> w245
              frame "Idle", Default {
                n74 = call <vilib>:"Unset Busy.vi"("error in (no error)"=w248) -> ("error out"=w247:errorcluster)  [unwired: 10 in]
              }
              frame "Busy" {
                n75 = call <vilib>:"Set Busy.vi"("error in (no error)"=w250) -> ("error out"=w249:errorcluster)  [unwired: 9 in, 1 out]
              }
            }
          }
          frame condition #1 {
          }
        }
        n76 = call <vilib>:"Add State(s) to Queue__JKI_lib_State_Machine.vi"("State(s) in (\"\")"=w243) -> ("States Out"=w242:string)  [unwired: 14 in]
      }
      frame "UI: Front Panel State" {
        # "Argument"
        # "Set Front Panel Open or Closed\n(Usage: \"UI: Front Panel State >> Open|Close\")"
        n77 = Unbundle By Name(w255) -> ("Core.Current VI Reference"=w254:refnum<vi>)
        n78 = call <vilib>:"Add State(s) to Queue__JKI_lib_State_Machine.vi"("State(s) in (\"\")"=w259) -> ("States Out"=w258:string)  [unwired: 14 in]
        n79 = case shown="\"Minimize\", \"Minimized\"" w253 {
          tunnel: w257 -> [w265 w280 w291 w304 w317]
          tunnel: [w267 w281 w293 w306 w319] -> w256
          tunnel: w254 -> [w266 w278 w292 w305 w318]
          frame "Open", "Standard", Default {
            w260 = T1."Standard" ("State")
            n80 = property class="VI"(reference=w266, error in=w265) -> (reference out=w263:refnum<vi>, error out=w264:errorcluster, "FP.State"=w262:T1)
            n81 = Not Equal?(x=w262, y=w260) -> (x != y?=w261:bool)
            n82 = case shown="True" w261 {
              tunnel: [w271 w273] -> w267
              tunnel: w264 -> [w270 w273]
              tunnel: w263 -> [w269 _]
              tunnel: w260 -> [w268 _]
              frame True {
                n83 = invoke class="VI" method="FP.Open"(reference=w269, error in=w270, "Activate"=TRUE, "State"=w268) -> (error out=w271:errorcluster)  [unwired: 1 in, 4 out]
              }
              frame False {
              }
            }
          }
          frame "Close", "Closed" {
            n84 = property class="VI"(reference=w278, error in=w280) -> (reference out=w277:refnum<vi>, error out=w279:errorcluster, "FP.State"=w275:T1)
            n85 = Not Equal?(x=w275, y=T1."Closed" ("Front Panel Window:State")) -> (x != y?=w274:bool)
            n86 = case shown="True" w274 {
              tunnel: [w282 w285] -> w281
              tunnel: w279 -> [w282 w284]
              tunnel: w277 -> [_ w283]
              frame False {
              }
              frame True {
                n87 = invoke class="VI" method="FP.Close"(reference=w283, error in=w284) -> (error out=w285:errorcluster)  [unwired: 1 in, 2 out]
              }
            }
          }
          frame "Hidden", "Hide" {
            w286 = T1."Hidden" ("State")
            n88 = property class="VI"(reference=w292, error in=w291) -> (reference out=w289:refnum<vi>, error out=w290:errorcluster, "FP.State"=w288:T1)
            n89 = Not Equal?(x=w288, y=w286) -> (x != y?=w287:bool)
            n90 = case shown="True" w287 {
              tunnel: [w297 w298] -> w293
              tunnel: w290 -> [w296 w298]
              tunnel: w289 -> [w295 _]
              tunnel: w286 -> [w294 _]
              frame True {
                n91 = invoke class="VI" method="FP.Open"(reference=w295, error in=w296, "State"=w294) -> (error out=w297:errorcluster)  [unwired: 2 in, 4 out]
              }
              frame False {
              }
            }
          }
          frame "Minimize", "Minimized" {
            w299 = T1."Minimized" ("State")
            n92 = property class="VI"(reference=w305, error in=w304) -> (reference out=w302:refnum<vi>, error out=w303:errorcluster, "FP.State"=w301:T1)
            n93 = Not Equal?(x=w301, y=w299) -> (x != y?=w300:bool)
            n94 = case shown="True" w300 {
              tunnel: [w310 w311] -> w306
              tunnel: w303 -> [w309 w311]
              tunnel: w302 -> [w308 _]
              tunnel: w299 -> [w307 _]
              frame True {
                n95 = invoke class="VI" method="FP.Open"(reference=w308, error in=w309, "State"=w307) -> (error out=w310:errorcluster)  [unwired: 2 in, 4 out]
              }
              frame False {
              }
            }
          }
          frame "Maximize", "Maximized" {
            w312 = T1."Maximized" ("State")
            n96 = property class="VI"(reference=w318, error in=w317) -> (reference out=w315:refnum<vi>, error out=w316:errorcluster, "FP.State"=w314:T1)
            n97 = Not Equal?(x=w314, y=w312) -> (x != y?=w313:bool)
            n98 = case shown="True" w313 {
              tunnel: [w323 w324] -> w319
              tunnel: w316 -> [w322 w324]
              tunnel: w315 -> [w321 _]
              tunnel: w312 -> [w320 _]
              frame True {
                n99 = invoke class="VI" method="FP.Open"(reference=w321, error in=w322, "State"=w320) -> (error out=w323:errorcluster)  [unwired: 2 in, 4 out]
              }
              frame False {
              }
            }
          }
        }
      }
      frame "---------- Macro ----------" {
        # "Do not put any code in this frame.\n(It is a separator no-op. You can make a copy of this frame to create a new Macro frame)"
        n100 = call <vilib>:"Add State(s) to Queue__JKI_lib_State_Machine.vi"("State(s) in (\"\")"=w329) -> ("States Out"=w328:string)  [unwired: 14 in]
      }
      frame "Macro: Initialize" {
        w331 = "Data: Initialize\nInitialize Core Data\nEvents: Register\nUI: Initialize\nUI: Front Panel State >> Open"  # Data: Initialize Initialize Core Data Events: Register UI: Initialize UI: Front Panel State >> Open
        # "Initialization Macro\n(This is called once, when the VI starts)"
        n101 = call <vilib>:"Add State(s) to Queue__JKI_lib_State_Machine.vi"("State(s) in Front (\"\")"=w331, "State(s) in (\"\")"=w335) -> ("States Out"=w334:string)  [unwired: 13 in]
      }
      frame "Macro: Exit" {
        # "Exit Macro\n(This is called once, when the VI exits)"
        n102 = Unbundle By Name(w343) -> ("Core.Close Panel on Exit?"=w342:bool)
        n103 = Select(t="UI: Front Panel State >> Close", s=w342, f="") -> (s? t:f=w339:string)
        n104 = call <vilib>:"Add State(s) to Queue__JKI_lib_State_Machine.vi"("State(s) in (\"\")"=w339, "State(s) at Back (\"\")"="Data: Cleanup\nEvents: Unregister\nExit") -> ("States Out"=w337:string)  [unwired: 13 in]
        n105 = call <vilib>:"Add State(s) to Queue__JKI_lib_State_Machine.vi"("State(s) in Front (\"\")"=w337, "State(s) in (\"\")"=w346) -> ("States Out"=w345:string)  [unwired: 13 in]
      }
      frame "---------- API ----------" {
        # "Do not put any code in this frame.\n(It is a separator no-op. This category is recommanded to use for external API)"
      }
      frame "API: API1" {
        # "If you need to tell who triggered this state , use this string. If it's this case itself, this string is \"\"."
        # "Deal with the parameter if any"
        # "Connect this to return the response of your API"
        # "Copy/Rename this case for your own API"
      }
      frame "API: API2" {
        # "unpack HexStr  to Variant\nif complex parameter is needed."
        # "Copy/Rename this case for your own API"
        n106 = call "JKISM++ Convert HexStr to Data.vi"("HEX String"=w357) -> ()  [unwired: 8 in, 1 out]
        n107 = disable-structure shown="Disabled" {
          disable-tunnel: [w362 "API2 Response"] -> w356
          frame Disabled {
            # "pack variant to hexstr \nif complex response is needed."
            # "complex Response"
            n108 = call "JKISM++ Convert Data to HexStr.vi"() -> ("HEX String (0-9,A-F)"=w362:string)  [unwired: 9 in]
          }
          frame Enabled {
          }
        }
      }
      frame "---------- DoSth ----------" {
        # "Template Separator\n(You can make a copy of, or modify, this frame)"
        n109 = call <vilib>:"Add State(s) to Queue__JKI_lib_State_Machine.vi"("State(s) in (\"\")"=w368) -> ("States Out"=w367:string)  [unwired: 14 in]
      }
      frame "DoSth: DoA" {
        # "Your code here.\n(You can make a copy of, or modify, this frame)"
        n110 = call <vilib>:"Add State(s) to Queue__JKI_lib_State_Machine.vi"("State(s) in (\"\")"=w374) -> ("States Out"=w373:string)  [unwired: 14 in]
      }
      frame "DoSth: DoB" {
        # "Your code here.\n(You can make a copy of, or modify, this frame)"
        n111 = call <vilib>:"Add State(s) to Queue__JKI_lib_State_Machine.vi"("State(s) in (\"\")"=w380) -> ("States Out"=w379:string)  [unwired: 14 in]
      }
    }
  }
  n112 = for {
    shift-right: [w381] -> w3
    shift-left: w4 -> [w386]
    tunnel: w1 -> [w385] mode=indexing
    n113 = call-by-ref "Wait On Asynchronous Call"(reference=w385, error in=w386) -> (reference out=w384:refnum<vi>, error out=w382:errorcluster)  [unwired: 12 in]
    n114 = invoke class="VI (strict)" method="FP.Close"(reference=w384, error in=w382) -> (error out=w383:errorcluster)  [unwired: 1 in, 2 out]
    n115 = call <vilib>:"Clear Errors.vi"("error in (no error)"=w383) -> ("error out"=w381:errorcluster)  [unwired: 6 in]
  }
  n116 = Close Reference(reference=w1, error in (no error)=w3) -> ()  [unwired: 1 out]
